vi "Read Prefix command.vi"(8 "error in (no error)":errorcluster, 11 "Keithley Meter in":refnum<class "Keithley Meter.lvclass">) -> (0 "error out":errorcluster, 2 "Prefix command":string, 3 "Keithley Meter out":refnum<class "Keithley Meter.lvclass">)   [LabVIEW 2015, in "Keithley Meter.lvclass"]
uses:
  Keithley Meter.lvclass
  Keithley Meter.lvclass/Keithley Meter.ctl
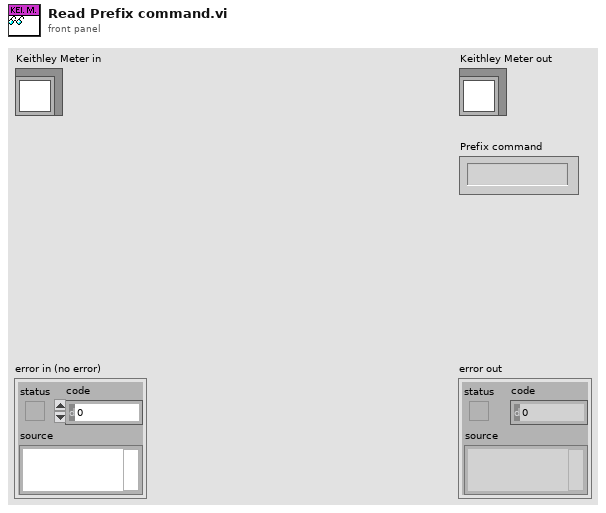
[diagram p1: front panel]
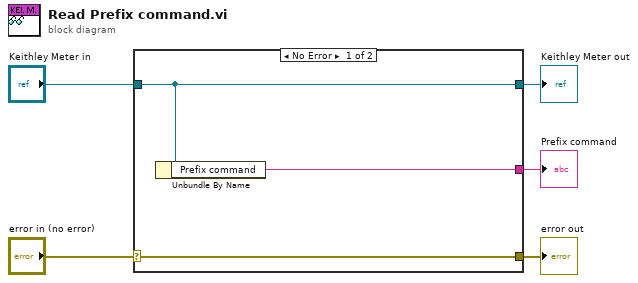
[diagram p0: block diagram]
diagram:
  n1 = case shown="No Error" "error in (no error)" {
    selector: "error in (no error)" -> [w8 w9]
    tunnel: [w8 w9] -> w4
    tunnel: [w7 w10] -> w2
    tunnel: "Keithley Meter in" -> [w7 w10]
    tunnel: [w6 _] -> w1
    frame No Error {
      n2 = Unbundle By Name(w7) -> ("Prefix command"=w6:string)
    }
    frame Error {
    }
  }
  "error out" <- w4
  "Keithley Meter out" <- w2
  "Prefix command" <- w1
